vi "authorize decode multi-part content.vi"(8 "error in (no error)":errorcluster, 10 "Valid Content-Type: (\"text/xml\")":string="text/xml", 11 "Multi-Part Content (\"\")":string) -> (0 "error out":errorcluster, 3 "Content":string)   [LabVIEW 2011]
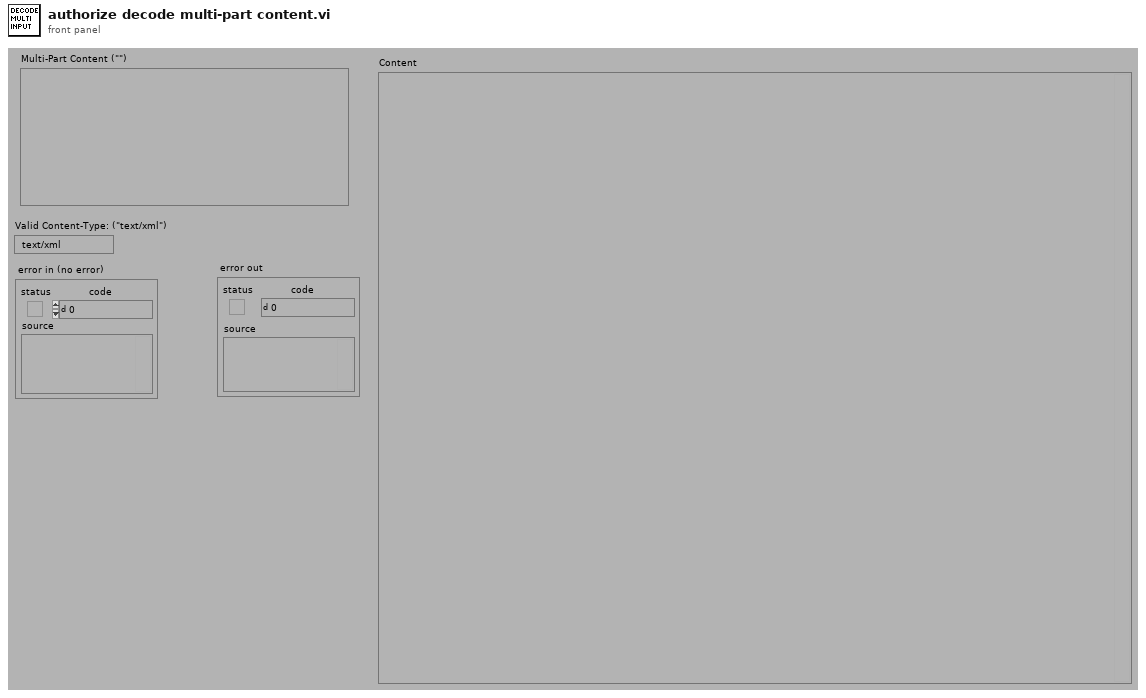
[diagram p1: front panel]
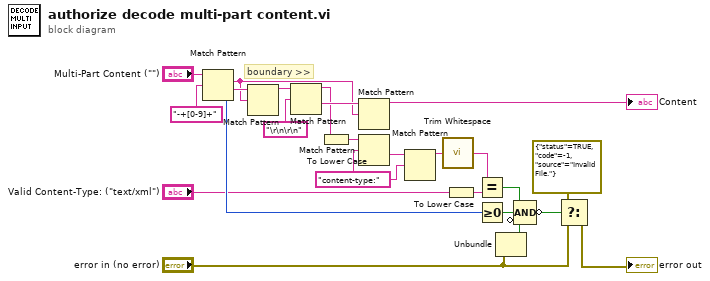
[diagram p0: block diagram]
diagram:
  w3 = "content-type:" ("regular expression")
  # "boundary >>"
  n1 = Match Pattern(string="Multi-Part Content (\"\")", regular expression="-+[0-9]+") -> (match substring=w6:string, after substring=w7:string, offset past match=w19:i32)  [unwired: 2 out]
  n2 = Match Pattern(string=w7, regular expression=w6) -> (before substring=w1:string)  [unwired: 4 out]
  n3 = Match Pattern(string=w1, regular expression="\r\n\r\n") -> (before substring=w5:string, after substring=w21:string)  [unwired: 3 out]
  n4 = To Lower Case(string=w5) -> (all lower case string=w9:string)
  n5 = Match Pattern(string=w21, regular expression=w6) -> (before substring=→"Content":string)  [unwired: 4 out]
  n6 = Match Pattern(string=w9, regular expression=w3) -> (after substring=w4:string)  [unwired: 4 out]
  n7 = Match Pattern(string=w4, regular expression=w3) -> (before substring=w2:string)  [unwired: 4 out]
  n8 = call <vilib>:"Trim Whitespace.vi"("string"=w2) -> ("trimmed string"=w8:string)  [unwired: 1 in]
  n9 = To Lower Case(string="Valid Content-Type: (\"text/xml\")") -> (all lower case string=w13:string)
  n10 = Equal?(x=w8, y=w13) -> (x = y?=w10:bool)
  n11 = Greater Or Equal To 0?(x=w19) -> (x >= 0?=w11:bool)
  n12 = Unbundle("error in (no error)") -> ("status"=w17:bool)  [unwired: 2 out]
  n13 = Compound Arithmetic op=AND(w10, w11, invert w17) -> (invert w18:bool)
  n14 = Select(t=errorcluster {"status"=TRUE, "code"=-1, "source"="Invalid File."}, s=w18, f="error in (no error)") -> (s? t:f=→"error out":errorcluster)
